vi "SecundsToH-M.vi"() -> ()   [LabVIEW 2023]
panel:
  in  "stop":bool
  out "Minutes":dbl
  out "Hour":dbl
  in  "Secunds":dbl
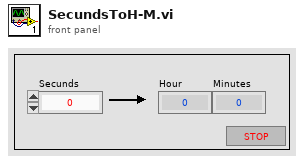
[diagram p1: front panel]
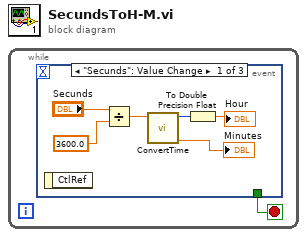
[diagram p0: block diagram]
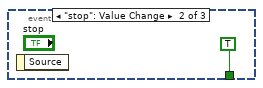
[diagram p2: hidden frame]
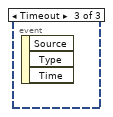
[diagram p3: hidden frame]
diagram:
  n1 = while {
    stop <- w1 stop-if-true
    n2 = event shown="[0] \"Secunds\": Value Change" {
      selector: _ -> [_ _ _]
      dyn-events: _ -> [_ _ _]
      timeout: _ -> [_ _ _]
      tunnel: [_ TRUE ("stop") _] -> w1
      event "Secunds": Value Change {
        n3 = event-data() -> ()  [unwired: 1 in, 1 out]
        n4 = Divide(x="Secunds", y=3600.0) -> (x/y=w2:dbl)
        n5 = call "ConvertTime.vi"("Час1"=w2) -> ("Минути"=→"Minutes":dbl, "Час"=w7:i64)  [unwired: 9 in]
        n6 = To Double Precision Float(number=w7) -> (double precision float=→"Hour":dbl)
      }
      event "stop": Value Change {
        n7 = event-data() -> ()  [unwired: 1 in, 1 out]
      }
      event Timeout {
        n8 = event-data() -> ()  [unwired: 1 in, 3 out]
      }
    }
  }
